vi "event_to_sub_focus.vi"(6 "interface":T1, 8 "error in (no error)":errorcluster) -> (0 "error out":errorcluster)   [LabVIEW 2015, in "lv-interface-sub-common.lvlib"]
uses:
  lv-interface-sub-common.lvlib
  _controls/interface_selection.ctl
  _controls/event_to_sub_command.ctl
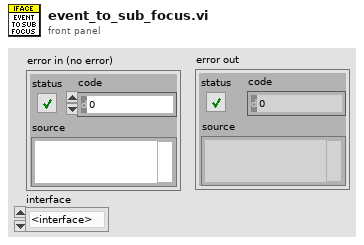
[diagram p1: front panel]
types:
  T1 = typedef "lv-interface-sub-common.lvlib/interface_selection.ctl" = enum16{"<interface>", "sub_interface_1", "sub_interface_2", "<null>"}
  T2 = typedef "lv-interface-sub-common.lvlib/event_to_sub_command.ctl" = enum16{"<to_sub_cmd>", "die", "focus", "unfocus", "<null>"}
  T3 = cluster{"command":T2, "interface":T1, "data":variant}
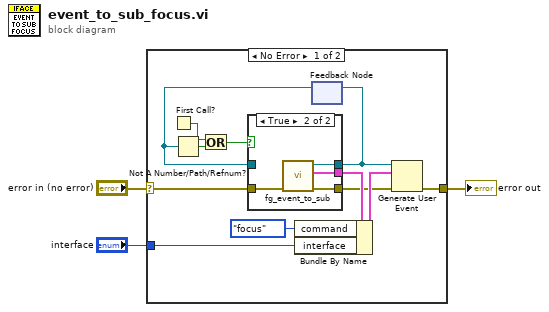
[diagram p0: block diagram]
diagram:
  n1 = case shown="No Error" "error in (no error)" {
    selector: "error in (no error)" -> [w15 w22]
    tunnel: [w10 w22] -> w2
    tunnel: "interface" -> [w4 _]
    frame No Error {
      n2 = First Call?() -> (First Call?: T/F=w6:bool)
      n3 = feedback #1() -> (w8:refnum<user-event>)  [unwired: 1 in]
      n4 = Not A Number/Path/Refnum?(number/path/refnum=w8) -> (NaN/Path/Refnum?=w7:bool)
      n5 = Or(x=w6, y=w7) -> (x .or. y?=w9:bool)
      n6 = case shown="True" w9 {
        tunnel: w15 -> [w16 w21]
        tunnel: [w17 w20] -> w14
        tunnel: [_ w19] -> w13
        tunnel: [w16 w18] -> w11
        tunnel: w8 -> [w17 _]
        frame False {
        }
        frame True {
          n7 = call "fg_event_to_sub.vi"("error in (no error)"=w21) -> ("error out"=w18:errorcluster, "data"=w19:T3, "to_sub"=w20:refnum<user-event>)  [unwired: 8 in]
        }
      }
      n8 = Bundle By Name(cluster=w13, "command"=event_to_sub_command."focus", "interface"=w4) -> (w12:T3)
      n9 = feedback-in #1(w14) -> ()
      n10 = Generate User Event(user event=w14, event data cluster=w12, error in=w11) -> (error out=w10:errorcluster)  [unwired: 1 in, 1 out]
    }
    frame Error {
    }
  }
  "error out" <- w2
